vi "RotationApplication.vi"() -> ()   [LabVIEW 2012]
uses:
  <instrlib>/ZaberTSeries/Public/Utility/Request.ctl
  <instrlib>/ZaberTSeries/Public/Utility/Response.ctl
  Event/MainEvents.ctl
  Event/AcquisitionEvents.ctl
  typedefs/Filenaming.ctl
  Spectrometer/Events/SpectrometerEvents.ctl
  Global/RotationGlobal.vi
  <vilib>/Utility/file.llb/Write To Spreadsheet File (string).vi
  variables/GlobalUI.vi
  Spectrometer/SpectrometerSpectraWiz.llb/StellarNet Globals.vi
  <instrlib>/ZaberTSeries/ZaberTSeries.lvlib
panel:
  in  "Rotation Speed deg/s":dbl=10.0
  in  "Sync Shotgun":bool
  in  "configuration file":path=path "C:/Users/Trent/Dropbox/Shared/Jeremy/microscoper 2012/ConfigFiles/Jeremy.ini"
  in  "Sync Data":bool=TRUE
  out "appended array":string[][](array[string])=[["theta (deg)", "0.000000", "1.000000", "2.000000", "3.000000", "4.000000", "5.000000", "6.000000", "7.000000", "8.000000", "9.000000", "10.000000", "11.000000", "12.000000", "13.000000", "14.000000", "15.000000", "16.000000", "17.000000", "18.000000", "19.000000", "20.000000", "21.000000", "22.000000", "23.000000", "24.000000", "25.000000", "26.000000", "27.000000", "28.000000", "29.000000", "30.000000", "31.000000", "32.000000", "33.000000", "34.000000", "35.000000", "36.000000", "37.000000", "38.000000", "39.000000", "40.000000", "41.000000", "42.000000", "43.000000", "44.000000", "45.000000"], ["77.0000", "0.0000", "0.0980", "0.1008", "0.1010", "0.0998", "0.1009", "0.1016", "0.1010", "0.1016", "0.1006", "0.0999", "0.1015", "0.1019", "0.1032", "0.1012", "0.1036", "0.1077", "0.1128", "0.1174", "0.1231", "0.1315", "0.1463", "0.1574", "0.1677", "0.1880", "0.2162", "0.2435", "0.3034", "0.4096", "0.4882", "0.5509", "0.5780", "0.6476", "0.7189", "0.6898", "0.6530", "0.6471", "0.6614", "0.6155", "0.6052", "0.6893", "0.6881", "0.6556", "0.7042", "0.7301", "0.7535"], ["77.1000", "0.7535", "0.1005", "0.1019", "0.1011", "0.1011", "0.1019", "0.1020", "0.1007", "0.1025", "0.1015", "0.0996", "0.1009", "0.0997", "0.0997", "0.0997", "0.1000", "0.1055", "0.1110", "0.1161", "0.1192", "0.1275", "0.1417", "0.1555", "0.1693", "0.1892", "0.2135", "0.2373", "0.2818", "0.3595", "0.4603", "0.5291", "0.5673", "0.6468", "0.7099", "0.6565", "0.6511", "0.6580", "0.5969", "0.6783", "0.6806", "0.6723", "0.6705", "0.7022", "0.7045", "0.7591", "0.9964"], ["77.2000", "0.9964", "0.0997", "0.0993", "0.1005", "0.1003", "0.1011", "0.0990", "0.1010", "0.1016", "0.1045", "0.1034", "0.1033", "0.1033", "0.1018", "0.1027", "0.1024", "0.1062", "0.1120", "0.1171", "0.1227", "0.1345", "0.1485", "0.1622", "0.1771", "0.1980", "0.2265", "0.2502", "0.2976", "0.3768", "0.4824", "0.5352", "0.5608", "0.6053", "0.6927", "0.7217", "0.6843", "0.6708", "0.6644", "0.6017", "0.6049", "0.6997", "0.6919", "0.7200", "0.8364", "0.8715", "0.9406"], ["77.3000", "0.9406", "0.1004", "0.1008", "0.0971", "0.0987", "0.1006", "0.1005", "0.1001", "0.0995", "0.1010", "0.1059", "0.1131", "0.1070", "0.1119", "0.1097", "0.1091", "0.1120", "0.1174", "0.1253", "0.1438", "0.1791", "0.2048", "0.2135", "0.2168", "0.2275", "0.2625", "0.2906", "0.3285", "0.4019", "0.5008", "0.5603", "0.5911", "0.6401", "0.7271", "0.7414", "0.7145", "0.6965", "0.6717", "0.6313", "0.7274", "0.7173", "0.7463", "0.8106", "0.9232", "1.0026", "1.1558"], ["77.4000", "1.1558", "0.0997", "0.1008", "0.1006", "0.1004", "0.0992", "0.1003", "0.1007", "0.1024", "0.1063", "0.1106", "0.1123", "0.1113", "0.1070", "0.1141", "0.1129", "0.1104", "0.1186", "0.1316", "0.1583", "0.1884", "0.2128", "0.2360", "0.2424", "0.2543", "0.2865", "0.3129", "0.3573", "0.4280", "0.5246", "0.5771", "0.5957", "0.6414", "0.7263", "0.7587", "0.7302", "0.7064", "0.6528", "0.7150", "0.7466", "0.7382", "0.7618", "0.8280", "0.9273", "1.0337", "1.1473"], ["77.5000", "1.1473", "0.1003", "0.0994", "0.0996", "0.0999", "0.0994", "0.1000", "0.1007", "0.1006", "0.1026", "0.1124", "0.1232", "0.1142", "0.1096", "0.1137", "0.1100", "0.1180", "0.1237", "0.1294", "0.1498", "0.1801", "0.2059", "0.2318", "0.2494", "0.2663", "0.2795", "0.3181", "0.3889", "0.4785", "0.5711", "0.5999", "0.6591", "0.7585", "0.7683", "0.7456", "0.7126", "0.7064", "0.6922", "0.6315", "0.7292", "0.7320", "0.7157", "0.7430", "0.7883", "0.8929", "0.9759"], ["77.6000", "0.9759", "0.0990", "0.1008", "0.1015", "0.1000", "0.0993", "0.0990", "0.1000", "0.1005", "0.1022", "0.1099", "0.1365", "0.1415", "0.1170", "0.1106", "0.1215", "0.1162", "0.1218", "0.1351", "0.1588", "0.1772", "0.1980", "0.2286", "", "", "", "", "", "", "", "", "", "", "", "", "", "", "", "", "", "", "", "", "", "", ""]]
  in  "Initialize":bool
  out "Angles (numeric)":dbl[](array[numeric])=[0.0, 1.0, 2.0, 3.0, 4.0, 5.0, 6.0, 7.0, 8.0, 9.0, 10.0, 11.0, 12.0, 13.0, 14.0, 15.0, 16.0, 17.0, 18.0, 19.0, 20.0, 21.0, 22.0, 23.0, 24.0, 25.0, 26.0, 27.0, 28.0, 29.0, 30.0, 31.0, 32.0, 33.0, 34.0, 35.0, 36.0, 37.0, 38.0, 39.0, 40.0, 41.0, 42.0, 43.0, 44.0, 45.0]
  out "Current angle pos":string[](array[string])=["77.6000", "0.9759", "0.0990", "0.1008", "0.1015", "0.1000", "0.0993", "0.0990", "0.1000", "0.1005", "0.1022", "0.1099", "0.1365", "0.1415", "0.1170", "0.1106", "0.1215", "0.1162", "0.1218", "0.1351", "0.1588", "0.1772", "0.1980", "0.2286"]
  out "Data":string[][](array[string])=[["theta (deg)", "0.000000", "1.000000", "2.000000", "3.000000", "4.000000", "5.000000", "6.000000", "7.000000", "8.000000", "9.000000", "10.000000", "11.000000", "12.000000", "13.000000", "14.000000", "15.000000", "16.000000", "17.000000", "18.000000", "19.000000", "20.000000", "21.000000", "22.000000", "23.000000", "24.000000", "25.000000", "26.000000", "27.000000", "28.000000", "29.000000", "30.000000", "31.000000", "32.000000", "33.000000", "34.000000", "35.000000", "36.000000", "37.000000", "38.000000", "39.000000", "40.000000", "41.000000", "42.000000", "43.000000", "44.000000", "45.000000"], ["77.0000", "0.0000", "0.0980", "0.1008", "0.1010", "0.0998", "0.1009", "0.1016", "0.1010", "0.1016", "0.1006", "0.0999", "0.1015", "0.1019", "0.1032", "0.1012", "0.1036", "0.1077", "0.1128", "0.1174", "0.1231", "0.1315", "0.1463", "0.1574", "0.1677", "0.1880", "0.2162", "0.2435", "0.3034", "0.4096", "0.4882", "0.5509", "0.5780", "0.6476", "0.7189", "0.6898", "0.6530", "0.6471", "0.6614", "0.6155", "0.6052", "0.6893", "0.6881", "0.6556", "0.7042", "0.7301", "0.7535"], ["77.1000", "0.7535", "0.1005", "0.1019", "0.1011", "0.1011", "0.1019", "0.1020", "0.1007", "0.1025", "0.1015", "0.0996", "0.1009", "0.0997", "0.0997", "0.0997", "0.1000", "0.1055", "0.1110", "0.1161", "0.1192", "0.1275", "0.1417", "0.1555", "0.1693", "0.1892", "0.2135", "0.2373", "0.2818", "0.3595", "0.4603", "0.5291", "0.5673", "0.6468", "0.7099", "0.6565", "0.6511", "0.6580", "0.5969", "0.6783", "0.6806", "0.6723", "0.6705", "0.7022", "0.7045", "0.7591", "0.9964"], ["77.2000", "0.9964", "0.0997", "0.0993", "0.1005", "0.1003", "0.1011", "0.0990", "0.1010", "0.1016", "0.1045", "0.1034", "0.1033", "0.1033", "0.1018", "0.1027", "0.1024", "0.1062", "0.1120", "0.1171", "0.1227", "0.1345", "0.1485", "0.1622", "0.1771", "0.1980", "0.2265", "0.2502", "0.2976", "0.3768", "0.4824", "0.5352", "0.5608", "0.6053", "0.6927", "0.7217", "0.6843", "0.6708", "0.6644", "0.6017", "0.6049", "0.6997", "0.6919", "0.7200", "0.8364", "0.8715", "0.9406"], ["77.3000", "0.9406", "0.1004", "0.1008", "0.0971", "0.0987", "0.1006", "0.1005", "0.1001", "0.0995", "0.1010", "0.1059", "0.1131", "0.1070", "0.1119", "0.1097", "0.1091", "0.1120", "0.1174", "0.1253", "0.1438", "0.1791", "0.2048", "0.2135", "0.2168", "0.2275", "0.2625", "0.2906", "0.3285", "0.4019", "0.5008", "0.5603", "0.5911", "0.6401", "0.7271", "0.7414", "0.7145", "0.6965", "0.6717", "0.6313", "0.7274", "0.7173", "0.7463", "0.8106", "0.9232", "1.0026", "1.1558"], ["77.4000", "1.1558", "0.0997", "0.1008", "0.1006", "0.1004", "0.0992", "0.1003", "0.1007", "0.1024", "0.1063", "0.1106", "0.1123", "0.1113", "0.1070", "0.1141", "0.1129", "0.1104", "0.1186", "0.1316", "0.1583", "0.1884", "0.2128", "0.2360", "0.2424", "0.2543", "0.2865", "0.3129", "0.3573", "0.4280", "0.5246", "0.5771", "0.5957", "0.6414", "0.7263", "0.7587", "0.7302", "0.7064", "0.6528", "0.7150", "0.7466", "0.7382", "0.7618", "0.8280", "0.9273", "1.0337", "1.1473"], ["77.5000", "1.1473", "0.1003", "0.0994", "0.0996", "0.0999", "0.0994", "0.1000", "0.1007", "0.1006", "0.1026", "0.1124", "0.1232", "0.1142", "0.1096", "0.1137", "0.1100", "0.1180", "0.1237", "0.1294", "0.1498", "0.1801", "0.2059", "0.2318", "0.2494", "0.2663", "0.2795", "0.3181", "0.3889", "0.4785", "0.5711", "0.5999", "0.6591", "0.7585", "0.7683", "0.7456", "0.7126", "0.7064", "0.6922", "0.6315", "0.7292", "0.7320", "0.7157", "0.7430", "0.7883", "0.8929", "0.9759"]]
  in  "VISA reference name:":refnum<visa-resource-name>="COM4"
  in  "OriginalFormula":string="+(0.00000000042880410878)*x*x*x*x*x*x*x*x*x*x*x+(-0.00000012876313032732)*x*x*x*x*x*x*x*x*x*x+(0.00001046910402408158)*x*x*x*x*x*x*x*x*x+(0.00027218428359585586)*x*x*x*x*x*x*x*x+(-0.04647428795671625784)*x*x*x*x*x*x*x+(-2.45256660925813374519)*x*x*x*x*x*x+(171.99232685775481854762)*x*x*x*x*x+(19228.38181468347102054395)*x*x*x*x+(-547735.32786055072210729122)*x*x*x+(-128477524.84194929897785186768)*x*x+(8402430653.59582424163818359375)*x+(-150659796088.04968261718750000000)"
  out "Current Angle (deg)":dbl=13.4634375
  out "Stage Position (mm)":dbl=92.62999725341797
  in  "Time Step (ms)":dbl=100.0
  in  "Stop":bool
  in  "Sync Formula":bool
  in  "Go Home":bool
  in  "Set Home Offset":dbl=83.8
  in  "TabControl":T1(tab)=enum."Stage Sync Data"
  in  "Optimize":bool
  in  "Move Rel +":bool
  in  "Move Abs?":bool
  in  "Move Rel (deg)":dbl=0.5 min=0.0 step=0.1
  in  "Move Abs (deg)":dbl=25.0
  in  "Send":bool
  in  "REQUEST:":T2={"Device Number"=1, "Command"=23, "Data"=-10000, "Response Count"=1} {"Command" items=["Echo"=55, "Home"=1, "Move Absolute"=20, "Move Relative"=21, "Move at Constant Speed"=22, "Renumber"=2, "Restore Settings"=36, "Stop"=23]}
  out "Response Data:":T3 {"Command" items=["Constant Speed Tracking"=8, "Echo"=55, "Error"=255, "Home"=1, "Limit Active"=9, "Manual Move Tracking"=10, "Move Absolute"=20, "Move at Constant Speed"=22, "Move Relative"=21, "Renumber"=2, "Restore Settings"=36, "Stop"=23]}
  in  "angle":dbl=12.0
  in  "Move Rel -":bool
  in  "reference data":path=path "C:/Users/Trent/Dropbox/Shared/Jeremy/Jeremy Shared Microscoper Data/rotCalib.csv"
  in  "Sync Speed (theta/s)":dbl=5.0
  in  "Formula File":path=path "C:/Users/Trent/Dropbox/Shared/Jeremy/Jeremy Shared Microscoper Data/calibrationformula.txt"
  in  "Rotation f(x) (mm -> deg)":string="+(0.6496827919)*x*x*x*x+(-203.4109451416)*x*x*x+(23882.0577216599)*x*x+(-1246170.6707626400)*x+(24383911.2035702057)"
  in  "Clear":bool
  in  "Final Angle":dbl=45.0
  in  "stop":bool
  out "Spectrum":T4(graph)
  in  "Step Size (deg) Surf1":dbl=0.5
  in  "Calibrate":bool
  in  "Get Data From PMT channel":i32=3
  in  "Aquire AngleScan":bool
  out "Intensity vs Angle Plot":cluster{"Angles (numeric)":dbl[], dbl[]}(graph)={"Angles (numeric)"=[0.0, 1.0, 2.0, 3.0, 4.0, 5.0, 6.0, 7.0, 8.0, 9.0, 10.0, 11.0, 12.0, 13.0, 14.0, 15.0, 16.0, 17.0, 18.0, 19.0, 20.0, 21.0, 22.0, 23.0, 24.0, 25.0, 26.0, 27.0, 28.0, 29.0, 30.0, 31.0, 32.0, 33.0, 34.0, 35.0, 36.0, 37.0, 38.0, 39.0, 40.0, 41.0, 42.0, 43.0, 44.0, 45.0], [0.9759, 0.099, 0.1008, 0.1015, 0.1, 0.0993, 0.099, 0.1, 0.1005, 0.1022, 0.1099, 0.1365, 0.1415, 0.117, 0.1106, 0.1215, 0.1162, 0.1218, 0.1351, 0.1588, 0.1772, 0.198, 0.2286]}
  in  "Step Size (deg)":dbl=1.0
  in  "Final Angle (deg)":dbl=45.0
  in  "Initial Angle (deg)":dbl
  out "AngleScanning?":bool
  out "File Destination":path=path "C:/Users/Trent/Documents/Jeremy/2016-10-24/ChixBone_8mW_190mW_700mV_700mV_700mV_6x_4ms_sf_00.csv"
  in  "Initialize AngleScan":bool
  in  "Save":bool=TRUE
  # "==>"
  # "Device"
  # "Command (Binary)"
  # "Data"
  # "==>"
  # "Data"
  # "==>"
  # "Rotation Mount Settings:"
  # "Simulated Delay Stage Settings:"
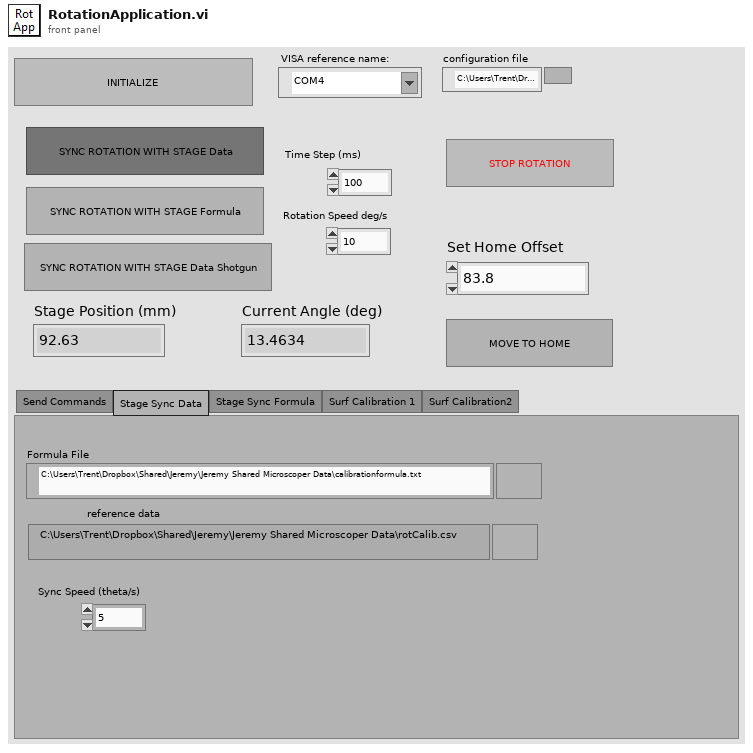
[diagram p1: front panel]
types:
  T1 = enum32{"Send Commands", "Stage Sync Data", "Stage Sync Formula", "Surf Calibration 1", "Surf Calibration2", "Simulated f(x)  ", "Adjust Simulation Settings"}
  T2 = typedef "ZaberTSeries.lvlib/Request.ctl" = cluster{"Device Number":u8, "Command":u8, "Data":i32, "Response Count":i32}
  T3 = typedef "ZaberTSeries.lvlib/Response.ctl" = cluster{"Device Number":u8, "Command":u8, "Data":i32}
  T4 = cluster{"Spectrometer wavelengths":sgl[], "buffer out":sgl[]}
  T5 = typedef "AcquisitionEvents.ctl" = enum16{"TimeOut", "Clear", "Acquire"}
  T6 = typedef "MainEvents.ctl" = enum16{"Initialize", "Initialize Angle Scan", "Acquire Angle Scan", "Move to Zero", "Home", "Send Request", "Move Relative Negative", "Move Relative", "Optimize", "Move Absolute", "Calibrate Angle-Stage", "Restore Sync Parameters", "Sync Formula", "Sync Data", "Sync Data Shotgun", "Restore Booleans", "Disable Buttons", "Enable Buttons"}
  T7 = typedef "SpectrometerEvents.ctl" = enum16{"TimeOut", "Init Programmatically", "Init Button", "Init Background", "Acquire Background", "Acquire"}
  T8 = enum8{"Enabled", "Disabled", "Disabled and Grayed Out"}
  T9 = typedef "Stage Parameters.ctl" = cluster{"Scan Mode":T10, "Start position mm":dbl, "End position mm":dbl, "Velocity um/sec (continuous)":dbl, "Step size microns (discrete)":dbl, "Frames to grab (grab)":i32}
  T10 = typedef "ScanMode.ctl" = enum16{"None", "Continuous", "Point Scan (CH3 cursor)", "Point Scan Move (CH3 cursor)", "Grab", "Grab Move Stage", "Grab Move Z-stage", "Cont. Move Z-stage", "Spec Move Stage", "Spec Move Cont", "Surf Calib"}
  T11 = typedef "Filenaming.ctl" = enum16{"Image", "Just Description"}
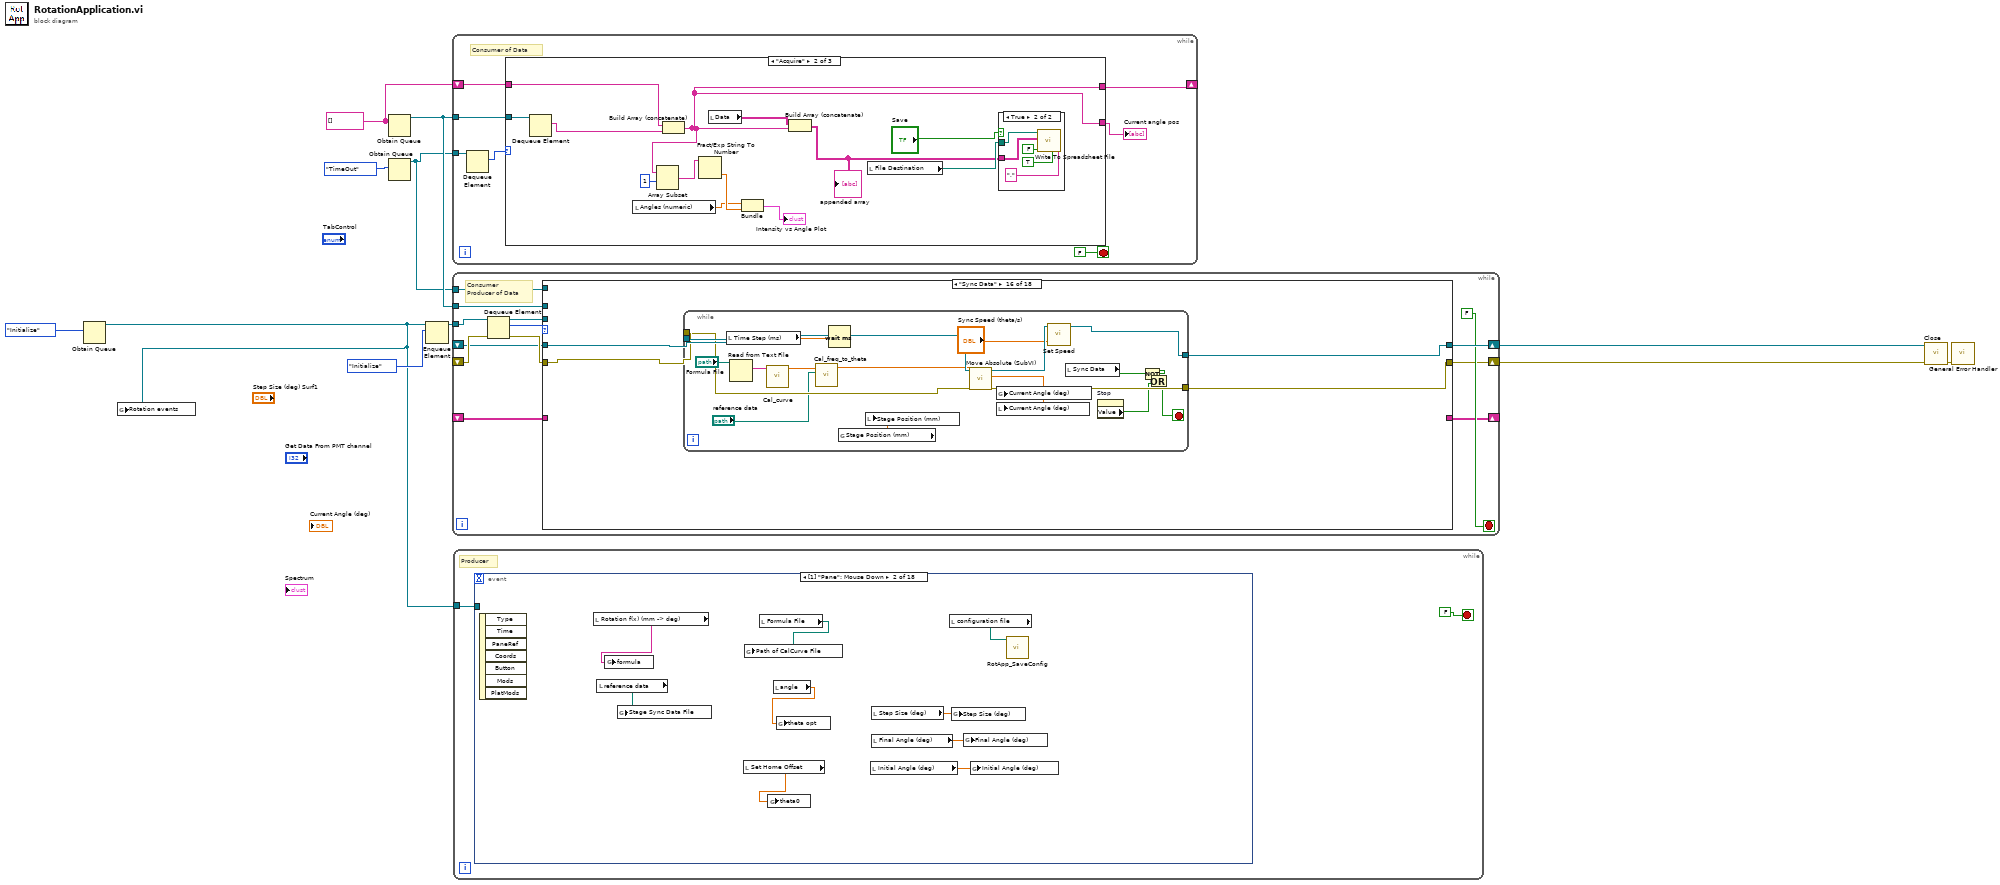
[diagram p0: block diagram]
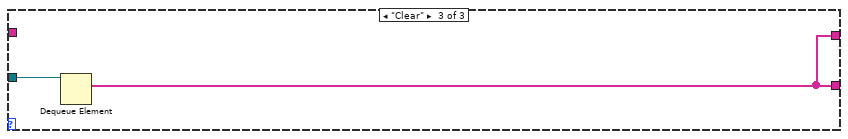
[diagram p4: hidden frame]
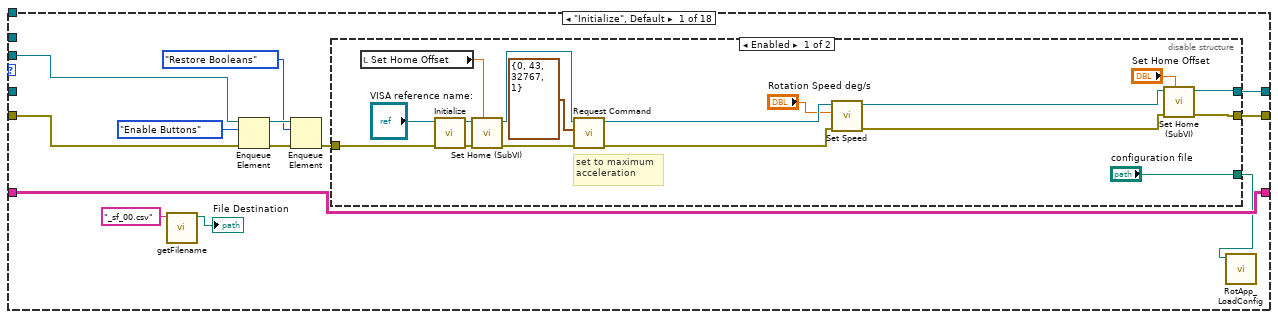
[diagram p5: hidden frame]
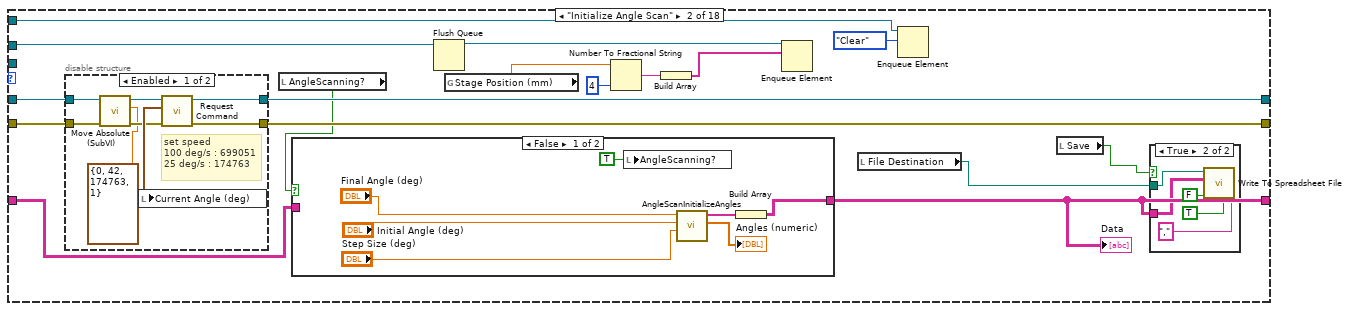
[diagram p7: hidden frame]
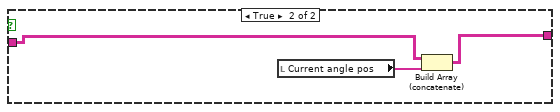
[diagram p9: hidden frame]
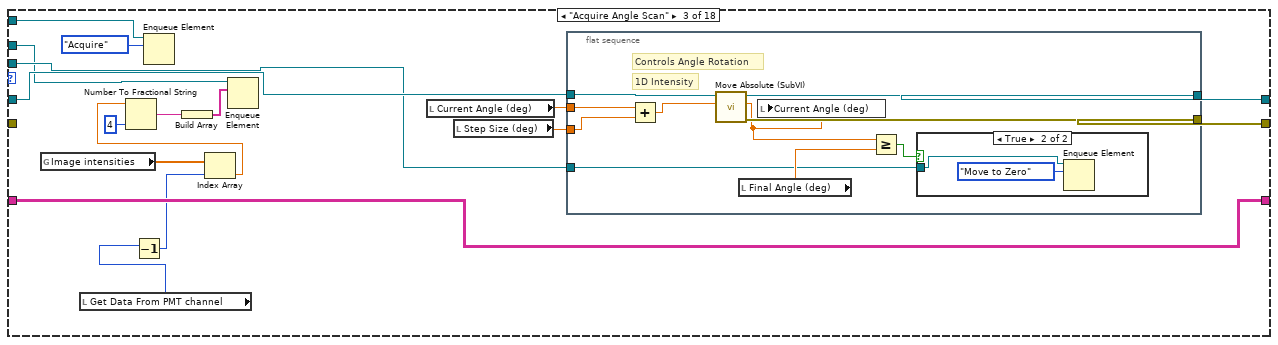
[diagram p11: hidden frame]
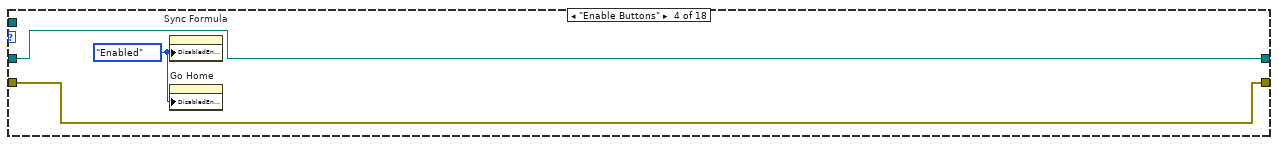
[diagram p13: hidden frame]
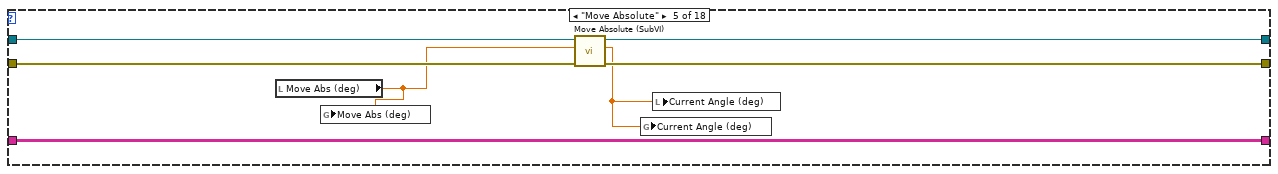
[diagram p14: hidden frame]
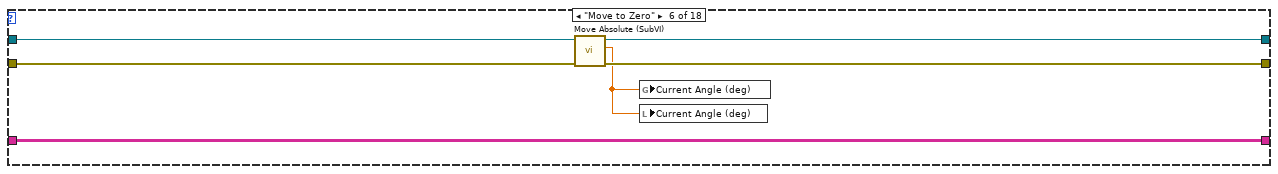
[diagram p15: hidden frame]
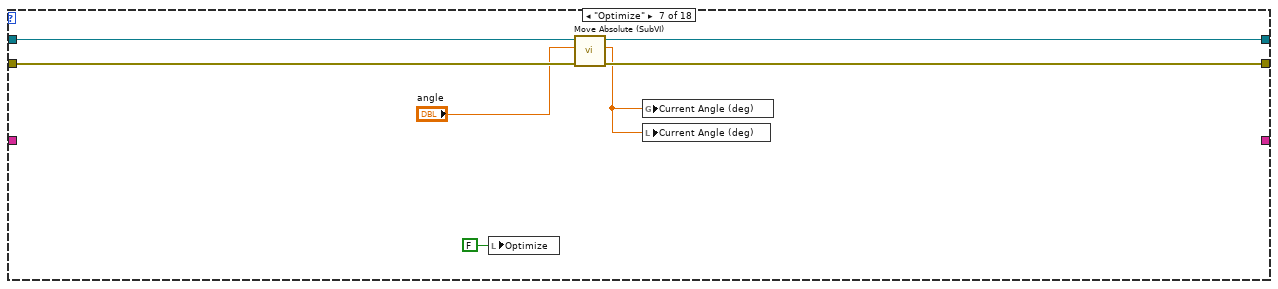
[diagram p16: hidden frame]
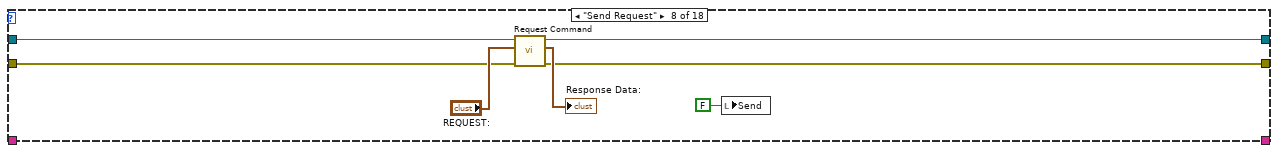
[diagram p17: hidden frame]
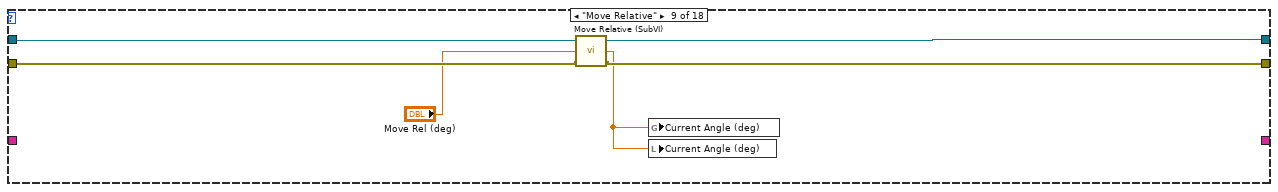
[diagram p18: hidden frame]
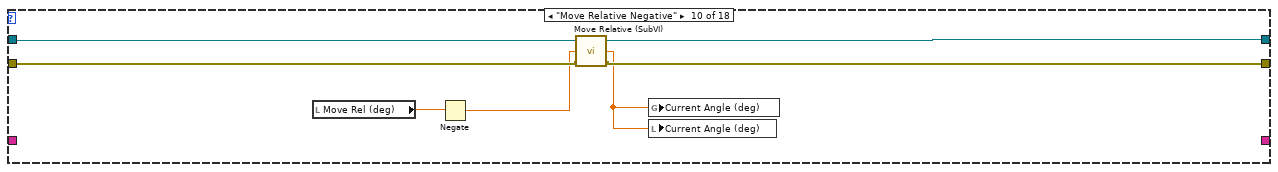
[diagram p19: hidden frame]
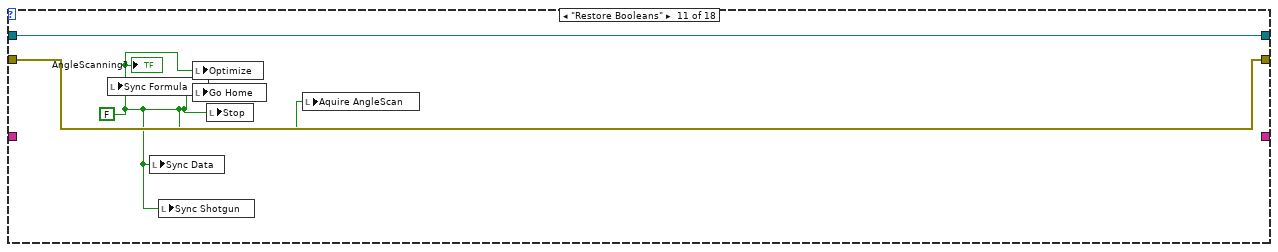
[diagram p20: hidden frame]
diagram:
  w4 = string[] []
  n1 = Obtain Queue(element data type=MainEvents."Initialize") -> (queue out=w1:refnum<queue>)  [unwired: 4 in, 2 out]
  n2 = global write "RotationGlobal.vi" "Rotation events"(w1) -> ()
  n3 = Obtain Queue(element data type=w4) -> (queue out=w5:refnum<queue>)  [unwired: 4 in, 2 out]
  n4 = Obtain Queue(element data type=AcquisitionEvents."TimeOut") -> (queue out=w2:refnum<queue>)  [unwired: 4 in, 2 out]
  n5 = Enqueue Element(queue=w1, element=MainEvents."Initialize") -> (queue out=w9:refnum<queue>)  [unwired: 2 in, 2 out]
  n6 = while {
    tunnel: w5 -> [w17]
    shift-right: [w13] -> _
    shift-left: w4 -> [w16]
    tunnel: w2 -> [w15]
    stop <- FALSE stop-if-true
    # "Consumer of Data"
    n7 = Dequeue Element(queue=w15) -> (element=w14:T5)  [unwired: 2 in, 3 out]
    n8 = case shown="\"Acquire\"" w14 {
      tunnel: w17 -> [_ w32 w39]
      tunnel: w16 -> [w19 w31 _]
      tunnel: [w19 w22 w38] -> w13
      tunnel: [w19 w22 w38] -> w12
      frame "TimeOut", Default {
      }
      frame "Acquire" {
        n9 = Dequeue Element(queue=w32) -> (element=w30:string[])  [unwired: 2 in, 3 out]
        n10 = local read "Angles (numeric)"() -> (w25:dbl[])
        n11 = Build Array (concatenate)(w31, w30) -> (w22:string[])
        n12 = Array Subset(array=w22, index=1) -> (w21:string[])  [unwired: 1 in]
        n13 = Fract/Exp String To Number(string=w21) -> (number=w26:dbl[])  [unwired: 3 in, 1 out]
        n14 = local read "Data"() -> (w27:string[][])
        n15 = Bundle("Angles (numeric)"=w25, w26) -> (→"Intensity vs Angle Plot":cluster{"Angles (numeric)":dbl[], dbl[]})  [unwired: 1 in]
        n16 = Build Array (concatenate)(w27, w22) -> (w28:string[][])
        "appended array" <- w28
        n17 = local read "File Destination"() -> (w29:path)
        n18 = case shown="True" "Save" {
          tunnel: w29 -> [_ w37]
          tunnel: w28 -> [_ w33]
          frame False {
          }
          frame True {
            n19 = call-poly <vilib>:"Write To Spreadsheet File.vi"("delimiter (\\t)"="," ("delimiter (\\t)"), "transpose? (no:F)"=TRUE, "append to file? (new file:F)"=FALSE, "2D data"=w33, "file path (dialog if empty)"=w37) -> ()  [unwired: 3 in, 1 out]
          }
        }
      }
      frame "Clear" {
        n20 = Dequeue Element(queue=w39) -> (element=w38:string[])  [unwired: 2 in, 3 out]
      }
    }
    "Current angle pos" <- w12
  }
  n21 = while {
    tunnel: w9 -> [w51]
    shift-right: [w50] -> w7
    shift-left: _ -> [w44]
    shift-right: [w47] -> w6
    shift-left: _ -> [w46]
    tunnel: w5 -> [w43]
    shift-right: [w42] -> _
    shift-left: _ -> [w41]
    tunnel: w2 -> [w40]
    stop <- FALSE stop-if-true
    # "Consumer\nProducer of Data"
    n22 = Dequeue Element(queue=w51, error in (no error)=w46) -> (queue out=w49:refnum<queue>, element=w52:T6, error out=w45:errorcluster)  [unwired: 1 in, 1 out]
    n23 = case shown="\"Sync Data\"" w52 {
      tunnel: [w65 w98 w141 w154 w163 w169 w176 w180 w189 w196 w198 w201 w205 w207 w211 w229 w250 w266] -> w50
      tunnel: w49 -> [w64 _ w127 _ _ _ _ _ _ _ _ _ _ _ _ _ _ w268]
      tunnel: [w58 w97 w138 w155 w161 w167 w174 w179 w187 w194 w199 w202 w204 w208 w213 w230 w252 w269] -> w47
      tunnel: w45 -> [w60 w99 _ w155 w162 w168 w175 w178 w188 w195 w199 w202 w206 w208 w212 w227 w251 w269]
      tunnel: w44 -> [_ w94 w129 w154 w160 w166 w171 w177 w185 w193 w198 w201 w203 w207 w210 w228 w249 w267]
      tunnel: w43 -> [_ w95 w126 _ _ _ _ _ _ _ _ _ _ _ _ _ _ _]
      tunnel: [w54 w90 w131 _ w159 w165 _ _ _ _ _ _ _ _ _ _ _ _] -> w42
      tunnel: w41 -> [w54 w93 w131 _ w159 w165 _ _ _ _ _ _ _ _ _ _ _ _]
      tunnel: w40 -> [_ w92 w132 _ _ _ _ _ _ _ _ _ _ _ _ _ _ _]
      frame "Initialize", Default {
        n24 = call "getFilename.vi"("Extension"="_sf_00.csv" ("string")) -> ("Filename"=→"File Destination":path)  [unwired: 10 in]
        n25 = Enqueue Element(queue=w64, element=MainEvents."Enable Buttons", error in (no error)=w60) -> (queue out=w62:refnum<queue>, error out=w59:errorcluster)  [unwired: 1 in, 1 out]
        n26 = Enqueue Element(queue=w62, element=MainEvents."Restore Booleans", error in (no error)=w59) -> (error out=w57:errorcluster)  [unwired: 1 in, 2 out]
        n27 = disable-structure shown="Enabled" {
          disable-tunnel: [w71 _] -> w65
          disable-tunnel: [w69 _] -> w58
          disable-tunnel: w57 -> [w82 _]
          disable-tunnel: ["configuration file" _] -> w53
          frame Enabled {
            # "set to maximum\nacceleration"
            n28 = local read "Set Home Offset"() -> (w67:dbl)
            n29 = call <instrlib>:"Initialize.vi"("error in (no error)"=w82, "VISA resource name"="VISA reference name:") -> ("error out"=w76:errorcluster, "VISA resource name out"=w75:refnum<visa-resource-name>)  [unwired: 7 in, 1 out]
            n30 = call "Set Home (SubVI).vi"("Home Offset (deg)"=w67, "error in (no error)"=w76, "VISA Refnum in"=w75) -> ("error out"=w78:errorcluster, "VISA Refnum out"=w77:refnum<visa-resource-name>)  [unwired: 7 in]
            n31 = call <instrlib>:"Request Command.vi"("error in (no error)"=w78, "Request"=T2 {"Device Number"=0, "Command"=43, "Data"=32767, "Response Count"=1}, "VISA resource name"=w77) -> ("error out"=w80:errorcluster, "VISA resource name out"=w79:refnum<visa-resource-name>)  [unwired: 5 in, 2 out]
            n32 = call "Set Speed.vi"("error in (no error)"=w80, "Rotation Speed deg/s"="Rotation Speed deg/s", "VISA Refnum in"=w79) -> ("error out"=w70:errorcluster, "VISA Refnum out"=w72:refnum<visa-resource-name>)  [unwired: 7 in]
            n33 = call "Set Home (SubVI).vi"("Home Offset (deg)"="Set Home Offset", "error in (no error)"=w70, "VISA Refnum in"=w72) -> ("error out"=w69:errorcluster, "VISA Refnum out"=w71:refnum<visa-resource-name>)  [unwired: 7 in]
          }
          frame Disabled {
          }
        }
        n34 = call "RotApp_LoadConfig.vi"("configuration file"=w53) -> ()  [unwired: 11 in]
      }
      frame "Initialize Angle Scan" {
        n35 = disable-structure shown="Enabled" {
          disable-tunnel: w99 -> [w122 w124]
          disable-tunnel: [w120 w123] -> w98
          disable-tunnel: [w119 w124] -> w97
          disable-tunnel: w94 -> [w116 w123]
          frame Enabled {
            # "set speed\n100 deg/s : 699051\n25 deg/s : 174763"
            n36 = call "Move Absolute (SubVI).vi"("error in (no error)"=w122, "VISA Refnum in"=w116) -> ("error out"=w117:errorcluster, "New Angle"=w115:dbl, "VISA Refnum out"=w118:refnum<visa-resource-name>)  [unwired: 7 in]
            n37 = local write "Current Angle (deg)"(w115) -> ()
            n38 = call <instrlib>:"Request Command.vi"("error in (no error)"=w117, "Request"=T2 {"Device Number"=0, "Command"=42, "Data"=174763, "Response Count"=1}, "VISA resource name"=w118) -> ("error out"=w119:errorcluster, "VISA resource name out"=w120:refnum<visa-resource-name>)  [unwired: 5 in, 2 out]
          }
          frame Disabled {
          }
        }
        n39 = local read "AngleScanning?"() -> (w96:bool)
        n40 = case shown="False" w96 {
          tunnel: [w106 w112] -> w90
          tunnel: w93 -> [_ w114]
          frame False {
            n41 = local write "AngleScanning?"(TRUE ("AngleScanning?")) -> ()
            n42 = call "AngleScanInitializeAngles.vi"("Step Size (deg)"="Step Size (deg)", "Initial Angle (deg)"="Initial Angle (deg)", "Final Angle (deg)"="Final Angle (deg)") -> ("Angles (numeric)"=→"Angles (numeric)":dbl[], "Angles (string)"=w107:string[])  [unwired: 7 in]
            n43 = Build Array(w107) -> (w106:string[][])
          }
          frame True {
            n44 = local read "Current angle pos"() -> (w113:string[])
            n45 = Build Array (concatenate)(w114, w113) -> (w112:string[][])
          }
        }
        "Data" <- w90
        n46 = Flush Queue(queue=w95) -> (queue out=w84:refnum<queue>)  [unwired: 1 in, 2 out]
        n47 = global read "GlobalUI.vi" "Stage Position (mm)"() -> (w85:dbl)
        n48 = Number To Fractional String(number=w85, precision (6)=i16 4) -> (F-format string=w86:string)  [unwired: 2 in]
        n49 = Build Array(w86) -> (w83:string[])
        n50 = Enqueue Element(queue=w84, element=w83) -> ()  [unwired: 2 in, 3 out]
        n51 = local read "File Destination"() -> (w88:path)
        n52 = Enqueue Element(queue=w92, element=AcquisitionEvents."Clear") -> ()  [unwired: 2 in, 3 out]
        n53 = local read "Save"() -> (w89:bool)
        n54 = case shown="True" w89 {
          tunnel: w88 -> [_ w104]
          tunnel: w90 -> [_ w101]
          frame False {
          }
          frame True {
            n55 = call-poly <vilib>:"Write To Spreadsheet File.vi"("delimiter (\\t)"="," ("delimiter (\\t)"), "transpose? (no:F)"=TRUE, "append to file? (new file:F)"=FALSE, "2D data"=w101, "file path (dialog if empty)"=w104) -> ()  [unwired: 3 in, 1 out]
          }
        }
      }
      frame "Acquire Angle Scan" {
        n56 = global read "GlobalUI.vi" "Image intensities"() -> (w137:dbl[])
        n57 = local read "Get Data From PMT channel"() -> (w125:i32)
        n58 = Decrement(x=w125) -> (x-1=w128:i32)
        n59 = Enqueue Element(queue=w132, element=AcquisitionEvents."Acquire") -> ()  [unwired: 2 in, 3 out]
        n60 = Index Array(array=w137, index=w128) -> (element=w130:dbl)
        n61 = Number To Fractional String(number=w130, precision (6)=i16 4) -> (F-format string=w135:string)  [unwired: 2 in]
        n62 = Build Array(w135) -> (w134:string[])
        n63 = Enqueue Element(queue=w126, element=w134) -> ()  [unwired: 2 in, 3 out]
        n64 = local read "Current Angle (deg)"() -> (w140:dbl)
        n65 = local read "Step Size (deg)"() -> (w139:dbl)
        n66 = flat-sequence {
          tunnel: [w151] -> w141
          tunnel: [w150] -> w138
          tunnel: w140 -> [w149]
          tunnel: w139 -> [w148]
          tunnel: w129 -> [w146]
          tunnel: w127 -> [w142]
          frame #0 {
            # "1D Intensity"
            # "Controls Angle Rotation"
            n67 = Add(x=w149, y=w148) -> (x+y=w147:dbl)
            n68 = call "Move Absolute (SubVI).vi"("Move to Angle"=w147, "VISA Refnum in"=w146) -> ("error out"=w150:errorcluster, "New Angle"=w145:dbl, "VISA Refnum out"=w151:refnum<visa-resource-name>)  [unwired: 7 in]
            n69 = local read "Final Angle (deg)"() -> (w144:dbl)
            n70 = local write "Current Angle (deg)"(w145) -> ()
            n71 = Greater Or Equal?(x=w145, y=w144) -> (x >= y?=w143:bool)
            n72 = case shown="True" w143 {
              tunnel: w142 -> [_ w153]
              frame False {
              }
              frame True {
                n73 = Enqueue Element(queue=w153, element=MainEvents."Move to Zero") -> ()  [unwired: 2 in, 3 out]
              }
            }
          }
        }
      }
      frame "Enable Buttons" {
        w156 = T8."Enabled" ("Disabled")
        n74 = property on="Sync Formula" class="Bool (strict)"("DisabledEnum"=w156) -> ()  [unwired: 2 in, 2 out]
        n75 = property on="Go Home" class="Bool (strict)"("DisabledEnum"=w156) -> ()  [unwired: 2 in, 2 out]
      }
      frame "Move Absolute" {
        n76 = local read "Move Abs (deg)"() -> (w157:dbl)
        n77 = global write "RotationGlobal.vi" "Move Abs (deg)"(w157) -> ()
        n78 = call "Move Absolute (SubVI).vi"("error in (no error)"=w162, "Move to Angle"=w157, "VISA Refnum in"=w160) -> ("error out"=w161:errorcluster, "New Angle"=w158:dbl, "VISA Refnum out"=w163:refnum<visa-resource-name>)  [unwired: 6 in]
        n79 = global write "RotationGlobal.vi" "Current Angle (deg)"(w158) -> ()
        n80 = local write "Current Angle (deg)"(w158) -> ()
      }
      frame "Move to Zero" {
        n81 = call "Move Absolute (SubVI).vi"("error in (no error)"=w168, "VISA Refnum in"=w166) -> ("error out"=w167:errorcluster, "New Angle"=w164:dbl, "VISA Refnum out"=w169:refnum<visa-resource-name>)  [unwired: 7 in]
        n82 = global write "RotationGlobal.vi" "Current Angle (deg)"(w164) -> ()
        n83 = local write "Current Angle (deg)"(w164) -> ()
      }
      frame "Optimize" {
        n84 = local write "Optimize"(FALSE ("Move Abs?")) -> ()
        n85 = call "Move Absolute (SubVI).vi"("error in (no error)"=w175, "Move to Angle"="angle", "VISA Refnum in"=w171) -> ("error out"=w174:errorcluster, "New Angle"=w170:dbl, "VISA Refnum out"=w176:refnum<visa-resource-name>)  [unwired: 6 in]
        n86 = global write "RotationGlobal.vi" "Current Angle (deg)"(w170) -> ()
        n87 = local write "Current Angle (deg)"(w170) -> ()
      }
      frame "Send Request" {
        n88 = call <instrlib>:"Request Command.vi"("error in (no error)"=w178, "Request"="REQUEST:", "VISA resource name"=w177) -> ("error out"=w179:errorcluster, "First Response"=→"Response Data:":T3, "VISA resource name out"=w180:refnum<visa-resource-name>)  [unwired: 5 in, 1 out]
        n89 = local write "Send"(FALSE ("Send")) -> ()
      }
      frame "Move Relative" {
        n90 = call "Move Relative (SubVI).vi"("error in (no error)"=w188, "Degrees to move"="Move Rel (deg)", "VISA resource name"=w185) -> ("error out"=w187:errorcluster, "New Angle"=w184:dbl, "VISA resource name out"=w189:refnum<visa-resource-name>)
        n91 = global write "RotationGlobal.vi" "Current Angle (deg)"(w184) -> ()
        n92 = local write "Current Angle (deg)"(w184) -> ()
      }
      frame "Move Relative Negative" {
        n93 = local read "Move Rel (deg)"() -> (w192:dbl)
        n94 = Negate(x=w192) -> (-x=w191:dbl)
        n95 = call "Move Relative (SubVI).vi"("error in (no error)"=w195, "Degrees to move"=w191, "VISA resource name"=w193) -> ("error out"=w194:errorcluster, "New Angle"=w190:dbl, "VISA resource name out"=w196:refnum<visa-resource-name>)
        n96 = global write "RotationGlobal.vi" "Current Angle (deg)"(w190) -> ()
        n97 = local write "Current Angle (deg)"(w190) -> ()
      }
      frame "Restore Booleans" {
        w197 = FALSE ("y")
        n98 = local write "Sync Formula"(w197) -> ()
        n99 = local write "Sync Data"(w197) -> ()
        n100 = local write "Sync Shotgun"(w197) -> ()
        n101 = local write "Optimize"(w197) -> ()
        n102 = local write "Go Home"(w197) -> ()
        n103 = local write "Stop"(w197) -> ()
        n104 = local write "Aquire AngleScan"(w197) -> ()
        "AngleScanning?" <- w197
      }
      frame "Restore Sync Parameters" {
        n105 = local write "Rotation f(x) (mm -> deg)"("" ("Rotation f(x) (mm -> deg)")) -> ()
      }
      frame "Home" {
        n106 = call "Go Home (SubVI).vi"("error in (no error)"=w206, "VISA Refnum in"=w203) -> ("error out"=w204:errorcluster, "VISA Refnum out"=w205:refnum<visa-resource-name>)  [unwired: 8 in]
      }
      frame "Disable Buttons" {
        w209 = T8."Disabled and Grayed Out" ("Disabled")
        n107 = property on="Sync Formula" class="Bool (strict)"("DisabledEnum"=w209) -> ()  [unwired: 2 in, 2 out]
        n108 = property on="Go Home" class="Bool (strict)"("DisabledEnum"=w209) -> ()  [unwired: 2 in, 2 out]
      }
      frame "Sync Formula" {
        n109 = while {
          tunnel: [w226] -> w211
          tunnel: [w225] -> w213
          tunnel: w212 -> [w220]
          tunnel: w210 -> [w217]
          stop <- w218 stop-if-true
          n110 = Wait (ms)(milliseconds to wait="Time Step (ms)") -> ()  [unwired: 1 out]
          n111 = call "Simple Function (SubVI).vi"("f(x) (mm -> deg)"="Rotation f(x) (mm -> deg)") -> ("Stage Position (mm)"=→"Stage Position (mm)":dbl, "Next Angle (deg)"=w223:dbl)  [unwired: 9 in]
          n112 = call "Move Absolute (SubVI).vi"("error in (no error)"=w220, "Move to Angle"=w223, "VISA Refnum in"=w217) -> ("error out"=w225:errorcluster, "New Angle"=w214:dbl, "VISA Refnum out"=w226:refnum<visa-resource-name>)  [unwired: 6 in]
          n113 = global write "RotationGlobal.vi" "Current Angle (deg)"(w214) -> ()
          n114 = local write "Current Angle (deg)"(w214) -> ()
          n115 = local read "Sync Formula"() -> (w216:bool)
          n116 = property on="Stop" class="Bool (strict)"() -> ("Value"=w219:bool)  [unwired: 2 in, 2 out]
          n117 = Not(x=w216) -> (.not. x?=w215:bool)
          n118 = Or(x=w215, y=w219) -> (x .or. y?=w218:bool)
        }
      }
      frame "Sync Data" {
        n119 = while {
          tunnel: [w234] -> w229
          tunnel: [w248] -> w230
          tunnel: w227 -> [w247]
          tunnel: w228 -> [w244]
          stop <- w245 stop-if-true
          n120 = local read "Time Step (ms)"() -> (w240:dbl)
          n121 = Read from Text File(file (use dialog)="Formula File") -> (text=w231:string)  [unwired: 3 in, 3 out]
          n122 = call "Cal_curve.vi"("Formula of Calibration Curve"=w231) -> ("Raman freq (cm-1)"=w239:dbl)  [unwired: 10 in]
          n123 = call "Cal_freq_to_theta.vi"("file path (dialog if empty)"="reference data", "Raman freq"=w239) -> ("predicted theta"=w237:dbl)  [unwired: 9 in]
          n124 = Wait (ms)(milliseconds to wait=w240) -> ()  [unwired: 1 out]
          n125 = global read "GlobalUI.vi" "Stage Position (mm)"() -> (w236:dbl)
          n126 = local write "Stage Position (mm)"(w236) -> ()
          n127 = call "Move Absolute (SubVI).vi"("error in (no error)"=w247, "Move to Angle"=w237, "VISA Refnum in"=w244) -> ("error out"=w248:errorcluster, "New Angle"=w241:dbl, "VISA Refnum out"=w235:refnum<visa-resource-name>)  [unwired: 6 in]
          n128 = global write "RotationGlobal.vi" "Current Angle (deg)"(w241) -> ()
          n129 = local write "Current Angle (deg)"(w241) -> ()
          n130 = call "Set Speed.vi"("Rotation Speed deg/s"="Sync Speed (theta/s)", "VISA Refnum in"=w235) -> ("VISA Refnum out"=w234:refnum<visa-resource-name>)  [unwired: 8 in, 1 out]
          n131 = local read "Sync Data"() -> (w243:bool)
          n132 = property on="Stop" class="Bool (strict)"() -> ("Value"=w246:bool)  [unwired: 2 in, 2 out]
          n133 = Not(x=w243) -> (.not. x?=w242:bool)
          n134 = Or(x=w242, y=w246) -> (x .or. y?=w245:bool)
        }
      }
      frame "Sync Data Shotgun" {
        n135 = while {
          tunnel: [w265] -> w250
          tunnel: [w264] -> w252
          tunnel: w251 -> [w263]
          tunnel: w249 -> [w260]
          stop <- w261 stop-if-true
          n136 = local read "Time Step (ms)"() -> (w256:dbl)
          n137 = local read "reference data"() -> (w254:path)
          n138 = call "Cal_stage_to_theta.vi"("file path (dialog if empty)"=w254) -> ("predicted theta"=w255:dbl)  [unwired: 10 in]
          n139 = global read "GlobalUI.vi" "Stage Position (mm)"() -> (w253:dbl)
          n140 = Wait (ms)(milliseconds to wait=w256) -> ()  [unwired: 1 out]
          n141 = local write "Stage Position (mm)"(w253) -> ()
          n142 = call "Move Absolute (SubVI).vi"("error in (no error)"=w263, "Move to Angle"=w255, "VISA Refnum in"=w260) -> ("error out"=w264:errorcluster, "New Angle"=w257:dbl, "VISA Refnum out"=w265:refnum<visa-resource-name>)  [unwired: 6 in]
          n143 = global write "RotationGlobal.vi" "Current Angle (deg)"(w257) -> ()
          n144 = local write "Current Angle (deg)"(w257) -> ()
          n145 = local read "Sync Shotgun"() -> (w259:bool)
          n146 = property on="Stop" class="Bool (strict)"() -> ("Value"=w262:bool)  [unwired: 2 in, 2 out]
          n147 = Not(x=w259) -> (.not. x?=w258:bool)
          n148 = Or(x=w258, y=w262) -> (x .or. y?=w261:bool)
        }
      }
      frame "Calibrate Angle-Stage" {
        n149 = disable-structure shown="Enabled" {
          disable-tunnel: w268 -> [_ w287]
          disable-tunnel: w267 -> [_ w286]
          disable-tunnel: [_ w285] -> w266
          frame Disabled {
            n150 = stacked-sequence {
              frame #0 {
                n151 = global read "GlobalUI.vi" "Stage Acquire Parameters"() -> (w280:T9)
                n152 = Unbundle By Name(w280) -> ("Start position mm"=w279:dbl, "End position mm"=w278:dbl)
                n153 = formula code="float64 m,b;\nm = 45/(xf-xi);\nb = -m*xi;"("xf"=w278, "xi"=w279) -> ("m"=w276:dbl, "b"=w277:dbl)
                n154 = local read "Rotation f(x) (mm -> deg)"() -> (w271:string)
                n155 = Format Into String(w276) -> (resulting string=w275:string)  [unwired: 3 in, 1 out]
                n156 = Format Into String(w277) -> (resulting string=w274:string)  [unwired: 3 in, 1 out]
                n157 = Concatenate Strings(w275, "*x + " ("string"), w274) -> (w270:string)
                n158 = Not Equal?(x=w271, y=w270) -> (x != y?=w272:bool)
                n159 = case shown="True" w272 {
                  tunnel: w271 -> [_ w282]
                  tunnel: w270 -> [_ w281]
                  frame False {
                  }
                  frame True {
                    n160 = stacked-sequence {
                      tunnel: w282 -> [w283 _]
                      tunnel: w281 -> [_ w284]
                      frame #0 {
                        n161 = local write "OriginalFormula"(w283) -> ()
                      }
                      frame #1 {
                        n162 = local write "Rotation f(x) (mm -> deg)"(w284) -> ()
                      }
                    }
                  }
                }
              }
            }
          }
          frame Enabled {
            n163 = global read "StellarNet Globals.vi" "SpectraWiz Events"() -> (w288:refnum<queue>)
            n164 = stacked-sequence {
              tunnel: w288 -> [w291 _ _ w297 w301]
              tunnel: w287 -> [_ _ _ _ w300]
              tunnel: w286 -> [_ w293 _ _ w303]
              tunnel: [_ _ _ _ w302] -> w285
              frame #0 {
                n165 = Enqueue Element(queue=w291, element=SpectrometerEvents."Init Programmatically") -> ()  [unwired: 2 in, 3 out]
                n166 = global read "GlobalUI.vi" "Stage Position (mm)"() -> (w289:dbl)
                n167 = local write "Stage Position (mm)"(w289) -> ()
              }
              frame #1 {
                n168 = call "Move Absolute (SubVI).vi"("VISA Refnum in"=w293) -> ("New Angle"=w292:dbl)  [unwired: 8 in, 2 out]
                n169 = global write "RotationGlobal.vi" "Current Angle (deg)"(w292) -> ()
                n170 = local write "Current Angle (deg)"(w292) -> ()
                n171 = Wait (ms)(milliseconds to wait=u32 2000) -> ()  [unwired: 1 out]
              }
              frame #2 {
                n172 = local read "Current Angle (deg)"() -> (w295:dbl)
                n173 = global write "GlobalUI.vi" "Stage Position (mm)"(w295) -> ()
              }
              frame #3 {
                n174 = Enqueue Element(queue=w297, element=SpectrometerEvents."Acquire") -> ()  [unwired: 2 in, 3 out]
                n175 = global write "StellarNet Globals.vi" "Scan OK"(FALSE ("Scan OK")) -> ()
                n176 = while {
                  stop <- w299 stop-if-true
                  n177 = global read "StellarNet Globals.vi" "Scan OK"() -> (w299:bool)
                }
              }
              frame #4 {
                n178 = while {
                  tunnel: w303 -> [w317]
                  tunnel: [w316] -> w302
                  tunnel: w301 -> [w315]
                  tunnel: w300 -> [w314]
                  stop <- w305 stop-if-true
                  # "Controls Angle Rotation"
                  n179 = local read "Current Angle (deg)"() -> (w311:dbl)
                  n180 = local read "Step Size (deg) Surf1"() -> (w310:dbl)
                  n181 = global write "GlobalUI.vi" "Stage Position (mm)"(w311) -> ()
                  n182 = Add(x=w311, y=w310) -> (x+y=w313:dbl)
                  n183 = global read "StellarNet Globals.vi" "Spectrum"() -> (w309:T4)
                  n184 = local write "Spectrum"(w309) -> ()
                  n185 = call "Move Absolute (SubVI).vi"("Move to Angle"=w313, "VISA Refnum in"=w317) -> ("New Angle"=w312:dbl, "VISA Refnum out"=w316:refnum<visa-resource-name>)  [unwired: 7 in, 1 out]
                  n186 = local write "Current Angle (deg)"(w312) -> ()
                  n187 = global write "StellarNet Globals.vi" "Scan OK"(FALSE ("Scan OK")) -> ()
                  n188 = Greater Or Equal?(x=w312, y="Final Angle") -> (x >= y?=w307:bool)
                  n189 = Or(x=w307, y="stop") -> (x .or. y?=w305:bool)
                  n190 = case shown="True" w307 {
                    tunnel: w315 -> [w318 _]
                    tunnel: w314 -> [_ w322]
                    frame False {
                      n191 = while {
                        stop <- w320 stop-if-true
                        n192 = global read "StellarNet Globals.vi" "Scan OK"() -> (w320:bool)
                      }
                      n193 = Enqueue Element(queue=w318, element=SpectrometerEvents."Acquire") -> ()  [unwired: 2 in, 3 out]
                    }
                    frame True {
                      n194 = Enqueue Element(queue=w322, element=MainEvents."Move to Zero") -> ()  [unwired: 2 in, 3 out]
                      n195 = local read "Stage Position (mm)"() -> (w321:dbl)
                      n196 = global write "GlobalUI.vi" "Stage Position (mm)"(w321) -> ()
                    }
                  }
                }
              }
            }
          }
        }
      }
    }
  }
  n197 = while {
    tunnel: w1 -> [w324]
    stop <- FALSE stop-if-true
    # "Producer"
    n198 = event shown="[1] \"Pane\": Mouse Down" {
      selector: _ -> [_ _ _ _ _ _ _ _ _ _ _ _ _ _ _ _ _ _]
      dyn-events: _ -> [_ _ _ _ _ _ _ _ _ _ _ _ _ _ _ _ _ _]
      timeout: _ -> [_ _ _ _ _ _ _ _ _ _ _ _ _ _ _ _ _ _]
      tunnel: w324 -> [_ _ w341 w345 w348 w353 w357 w361 w365 w369 w373 w377 _ w382 w384 w388 w394 w398]
      event Timeout {
        n199 = event-data() -> ()  [unwired: 1 in, 2 out]
      }
      event Mouse Down {
        n200 = event-data() -> ()  [unwired: 1 in, 7 out]
        n201 = local read "Rotation f(x) (mm -> deg)"() -> (w333:string)
        n202 = local read "reference data"() -> (w334:path)
        n203 = global write "RotationGlobal.vi" "formula"(w333) -> ()
        n204 = global write "RotationGlobal.vi" "Stage Sync Data File"(w334) -> ()
        n205 = local read "Set Home Offset"() -> (w330:dbl)
        n206 = local read "Formula File"() -> (w326:path)
        n207 = global write "RotationGlobal.vi" "Path of CalCurve File"(w326) -> ()
        n208 = global write "RotationGlobal.vi" "theta0"(w330) -> ()
        n209 = local read "angle"() -> (w331:dbl)
        n210 = global write "RotationGlobal.vi" "theta opt"(w331) -> ()
        n211 = local read "Initial Angle (deg)"() -> (w327:dbl)
        n212 = local read "Step Size (deg)"() -> (w329:dbl)
        n213 = local read "Final Angle (deg)"() -> (w328:dbl)
        n214 = local read "configuration file"() -> (w332:path)
        n215 = global write "RotationGlobal.vi" "Step Size (deg)"(w329) -> ()
        n216 = global write "RotationGlobal.vi" "Final Angle (deg)"(w328) -> ()
        n217 = global write "RotationGlobal.vi" "Initial Angle (deg)"(w327) -> ()
        n218 = call "RotApp_SaveConfig.vi"("configuration file"=w332) -> ()  [unwired: 11 in]
      }
      event "Calibrate": Value Change {
        (unwired) ""
        n219 = event-data() -> ()  [unwired: 1 in, 5 out]
        n220 = disable-structure shown="Enabled" {
          disable-tunnel: w341 -> [w342 _]
          frame Enabled {
            n221 = Enqueue Element(queue=w342, element=MainEvents."Calibrate Angle-Stage") -> ()  [unwired: 2 in, 3 out]
          }
          frame Disabled {
          }
        }
        n222 = global read "StellarNet Globals.vi" "Integration Time (ms)"() -> (w340:i32)
        n223 = Number To Fractional String(number=w340) -> (F-format string=w338:string)  [unwired: 3 in]
        n224 = global write "GlobalUI.vi" "Filenaming Mode"(Filenaming."Just Description" ("Filenaming Mode")) -> ()
        n225 = Concatenate Strings("SurfCal1_" ("Sample Description"), w338, "ms" ("string")) -> (w336:string)
        n226 = global write "GlobalUI.vi" "Sample Description"(w336) -> ()
      }
      event "Move Abs?": Value Change {
        n227 = event-data() -> ()  [unwired: 1 in, 5 out]
        n228 = case shown="True" "Move Abs?" {
          tunnel: w345 -> [_ w347]
          frame False {
          }
          frame True {
            n229 = Enqueue Element(queue=w347, element=MainEvents."Move Absolute") -> ()  [unwired: 2 in, 3 out]
          }
        }
      }
      event "Optimize": Value Change {
        n230 = event-data() -> ()  [unwired: 1 in, 5 out]
        n231 = case shown="True" "Optimize" {
          tunnel: w348 -> [_ w350]
          frame False {
          }
          frame True {
            n232 = Enqueue Element(queue=w350, element=MainEvents."Optimize") -> ()  [unwired: 2 in, 3 out]
          }
        }
      }
      event "Move Rel +": Value Change {
        n233 = event-data() -> ()  [unwired: 1 in, 5 out]
        n234 = case shown="True" "Move Rel +" {
          tunnel: w353 -> [_ w354]
          frame False {
          }
          frame True {
            n235 = Enqueue Element(queue=w354, element=MainEvents."Move Relative") -> ()  [unwired: 2 in, 3 out]
          }
        }
      }
      event "Move Rel -": Value Change {
        n236 = event-data() -> ()  [unwired: 1 in, 5 out]
        n237 = case shown="True" "Move Rel -" {
          tunnel: w357 -> [_ w358]
          frame False {
          }
          frame True {
            n238 = Enqueue Element(queue=w358, element=MainEvents."Move Relative Negative") -> ()  [unwired: 2 in, 3 out]
          }
        }
      }
      event "Send": Value Change {
        n239 = event-data() -> ()  [unwired: 1 in, 5 out]
        n240 = case shown="True" "Send" {
          tunnel: w361 -> [_ w362]
          frame False {
          }
          frame True {
            n241 = Enqueue Element(queue=w362, element=MainEvents."Send Request") -> ()  [unwired: 2 in, 3 out]
          }
        }
      }
      event "Initialize AngleScan": Value Change {
        n242 = event-data() -> ()  [unwired: 1 in, 5 out]
        n243 = case shown="True" "Initialize AngleScan" {
          tunnel: w365 -> [_ w366]
          frame False {
          }
          frame True {
            n244 = Enqueue Element(queue=w366, element=MainEvents."Initialize Angle Scan") -> ()  [unwired: 2 in, 3 out]
          }
        }
      }
      event "Go Home": Value Change {
        n245 = event-data() -> ()  [unwired: 1 in, 5 out]
        n246 = case shown="True" "Go Home" {
          tunnel: w369 -> [_ w370]
          frame False {
          }
          frame True {
            n247 = Enqueue Element(queue=w370, element=MainEvents."Home") -> ()  [unwired: 2 in, 3 out]
          }
        }
      }
      event "Aquire AngleScan": Value Change {
        n248 = event-data() -> ()  [unwired: 1 in, 5 out]
        n249 = case shown="True" "Aquire AngleScan" {
          tunnel: w373 -> [_ w374]
          frame False {
          }
          frame True {
            n250 = Enqueue Element(queue=w374, element=MainEvents."Acquire Angle Scan") -> ()  [unwired: 2 in, 3 out]
          }
        }
      }
      event "Initialize": Value Change {
        n251 = event-data() -> ()  [unwired: 1 in, 5 out]
        n252 = case shown="True" "Initialize" {
          tunnel: w377 -> [_ w378]
          frame False {
          }
          frame True {
            n253 = Enqueue Element(queue=w378, element=MainEvents."Initialize") -> ()  [unwired: 2 in, 3 out]
          }
        }
      }
      event "Move Abs (deg)": Value Change {
        n254 = event-data() -> ()  [unwired: 1 in, 5 out]
        n255 = global write "RotationGlobal.vi" "Move Abs (deg)"("Move Abs (deg)") -> ()
      }
      event "Clear": Value Change {
        n256 = event-data() -> ()  [unwired: 1 in, 5 out]
        n257 = Enqueue Element(queue=w382, element=MainEvents."Restore Sync Parameters") -> ()  [unwired: 2 in, 3 out]
      }
      event "Sync Formula": Value Change {
        n258 = event-data() -> ()  [unwired: 1 in, 5 out]
        n259 = case shown="True" "Sync Formula" {
          tunnel: w384 -> [_ w386]
          frame False {
          }
          frame True {
            n260 = Enqueue Element(queue=w386, element=MainEvents."Sync Formula") -> ()  [unwired: 2 in, 3 out]
          }
        }
      }
      event "Sync Data": Value Change {
        n261 = event-data() -> ()  [unwired: 1 in, 5 out]
        n262 = case shown="True" "Sync Data" {
          tunnel: w388 -> [_ w392]
          frame False {
          }
          frame True {
            n263 = Enqueue Element(queue=w392, element=MainEvents."Sync Data") -> (queue out=w390:refnum<queue>)  [unwired: 2 in, 2 out]
            n264 = Enqueue Element(queue=w390, element=MainEvents."Initialize") -> ()  [unwired: 2 in, 3 out]
          }
        }
      }
      event "Sync Shotgun": Value Change {
        n265 = event-data() -> ()  [unwired: 1 in, 5 out]
        n266 = case shown="True" "Sync Shotgun" {
          tunnel: w394 -> [_ w396]
          frame False {
          }
          frame True {
            n267 = Enqueue Element(queue=w396, element=MainEvents."Sync Data Shotgun") -> ()  [unwired: 2 in, 3 out]
          }
        }
      }
      event "Stop": Value Change {
        n268 = event-data() -> ()  [unwired: 1 in, 5 out]
        n269 = case shown="True" "Stop" {
          tunnel: w398 -> [_ w399]
          frame False {
          }
          frame True {
            n270 = Enqueue Element(queue=w399, element=MainEvents."Restore Booleans") -> ()  [unwired: 2 in, 3 out]
          }
        }
      }
    }
  }
  n271 = call <instrlib>:"Close.vi"("error in (no error)"=w6, "VISA resource name"=w7) -> ("error out"=w11:errorcluster)  [unwired: 8 in, 1 out]
  n272 = call <vilib>:"General Error Handler.vi"("error in (no error)"=w11) -> ()  [unwired: 10 in, 5 out]
